vi "End Session.vi"(8 "Error In":errorcluster, 11 "Reference In":i32) -> (0 "Error Out":errorcluster)   [LabVIEW 2009]
uses:
  Reference.vi
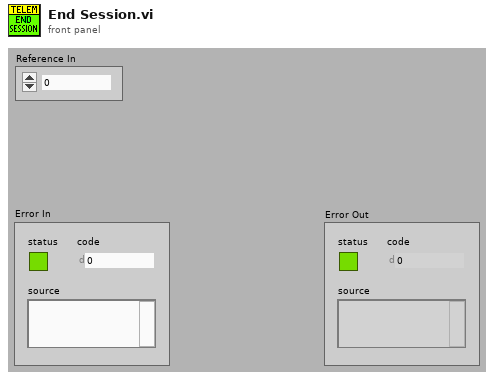
[diagram p1: front panel]
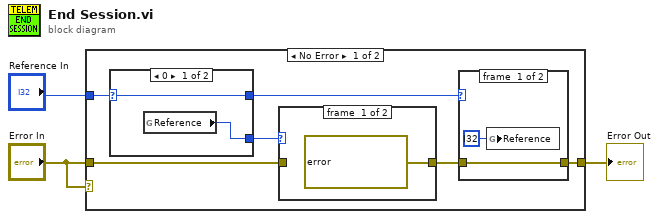
[diagram p0: block diagram]
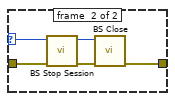
[diagram p2: hidden frame]
diagram:
  n1 = case shown="No Error" "Error In" {
    tunnel: "Error In" -> [w8 w22]
    tunnel: [w6 w22] -> w3
    tunnel: "Reference In" -> [w9 _]
    frame #0 {
      n2 = case shown="0" w9 {
        selector: w9 -> [w19 w21]
        tunnel: [w20 w21] -> w4
        tunnel: [w19 w21] -> w5
        frame #0 {
          n3 = global read "Reference.vi" "Reference"() -> (w20:i32)
        }
        frame #1 {
        }
      }
      n4 = case shown="1, Default" w4 {
        selector: w4 -> [_ w11]
        tunnel: w8 -> [_ w15]
        tunnel: [errorcluster ? ("Error Out") w12] -> w7
        frame #0 {
        }
        frame #1 {
          n5 = call <vilib>:"BS Stop Session.vi"("Error In"=w15, "Reference In"=w11) -> ("Error Out"=w14:errorcluster, "Reference Out"=w13:i32)  [unwired: 7 in]
          n6 = call <vilib>:"BS Close.vi"("Error In"=w14, "Reference In"=w13) -> ("Error Out"=w12:errorcluster)  [unwired: 7 in, 1 out]
        }
      }
      n7 = case shown="1, Default" w5 {
        tunnel: w7 -> [w17 w18]
        tunnel: [w17 w18] -> w6
        frame #0 {
          n8 = global write "Reference.vi" "Reference"(i32 ? ("Reference")) -> ()
        }
        frame #1 {
        }
      }
    }
    frame #1 {
    }
  }
  "Error Out" <- w3
